vi "KH TURCK ETHERNETIP IOL ByteToWord.vi"(11 "ByteArray":u8[](array[numeric])) -> (3 "WordArray":u16[](array[numeric]))   [LabVIEW 2021]
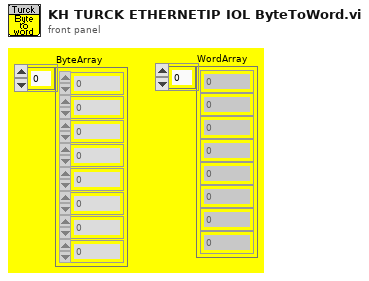
[diagram p1: front panel]
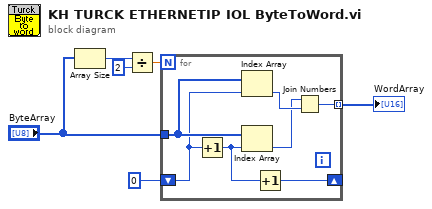
[diagram p0: block diagram]
diagram:
  n1 = Array Size(array="ByteArray") -> (size(s)=w4:i32)
  n2 = Divide(x=w4, y=2) -> (x/y=w1:dbl)
  n3 = for {
    N: w1 -> [_]
    tunnel: "ByteArray" -> [w11]
    tunnel: [w13] -> w2 mode=indexing
    shift-right: [w10] -> _
    shift-left: 0 -> [w9]
    n4 = Increment(x=w9) -> (x+1=w12:i32)
    n5 = Index Array(array=w11, index=w9) -> (element=w8:u8)
    n6 = Index Array(array=w11, index=w12) -> (element=w7:u8)
    n7 = Increment(x=w12) -> (x+1=w10:i32)
    n8 = Join Numbers(hi=w7, lo=w8) -> ((hi.lo)=w13:u16)
  }
  "WordArray" <- w2
